vi "Get Experiments from PGserver.vi"(6 "conninfo":T2={"host"="localhost", "port"="5432", "client_encoding"="WIN1251", "dbname"="data", "user"="postgres", "password"=""}, 8 "error in (no error)":errorcluster, 9 "ParamColumns":string[](array[string])=["N", "Description"], 10 "ParamTable":string="experiments_1") -> (0 "error out":errorcluster, 2 "Names table":string[][](array[string]), 3 "Parameters table":dbl[][](array[numeric]))   [LabVIEW 2019, in "control.lvlib"]
uses:
  control.lvlib
  Database/ctl/Coninfo.ctl
  Database/PostgreSQL2LabVIEW/libpqlv/src/PQfinish.vi
  Database/PostgreSQL2LabVIEW/libpqlv/src/PQconnectdb.vi
  Database/PostgreSQL2LabVIEW/libpqlv/src/PQerrorMessage.vi
  Database/PostgreSQL2LabVIEW/libpqlv/src/PQstatus.vi
  <vilib>/dlg_ctls.llb/Space Constant.vi
  Database/PostgreSQL2LabVIEW/libpqUtility64/libpqutility64.lvlib
  Database/PostgreSQL2LabVIEW/libpqUtility/libpqutility.lvlib
  Database/PostgreSQL.lvlib
panel:
  out "PQStatus":T1(ring)
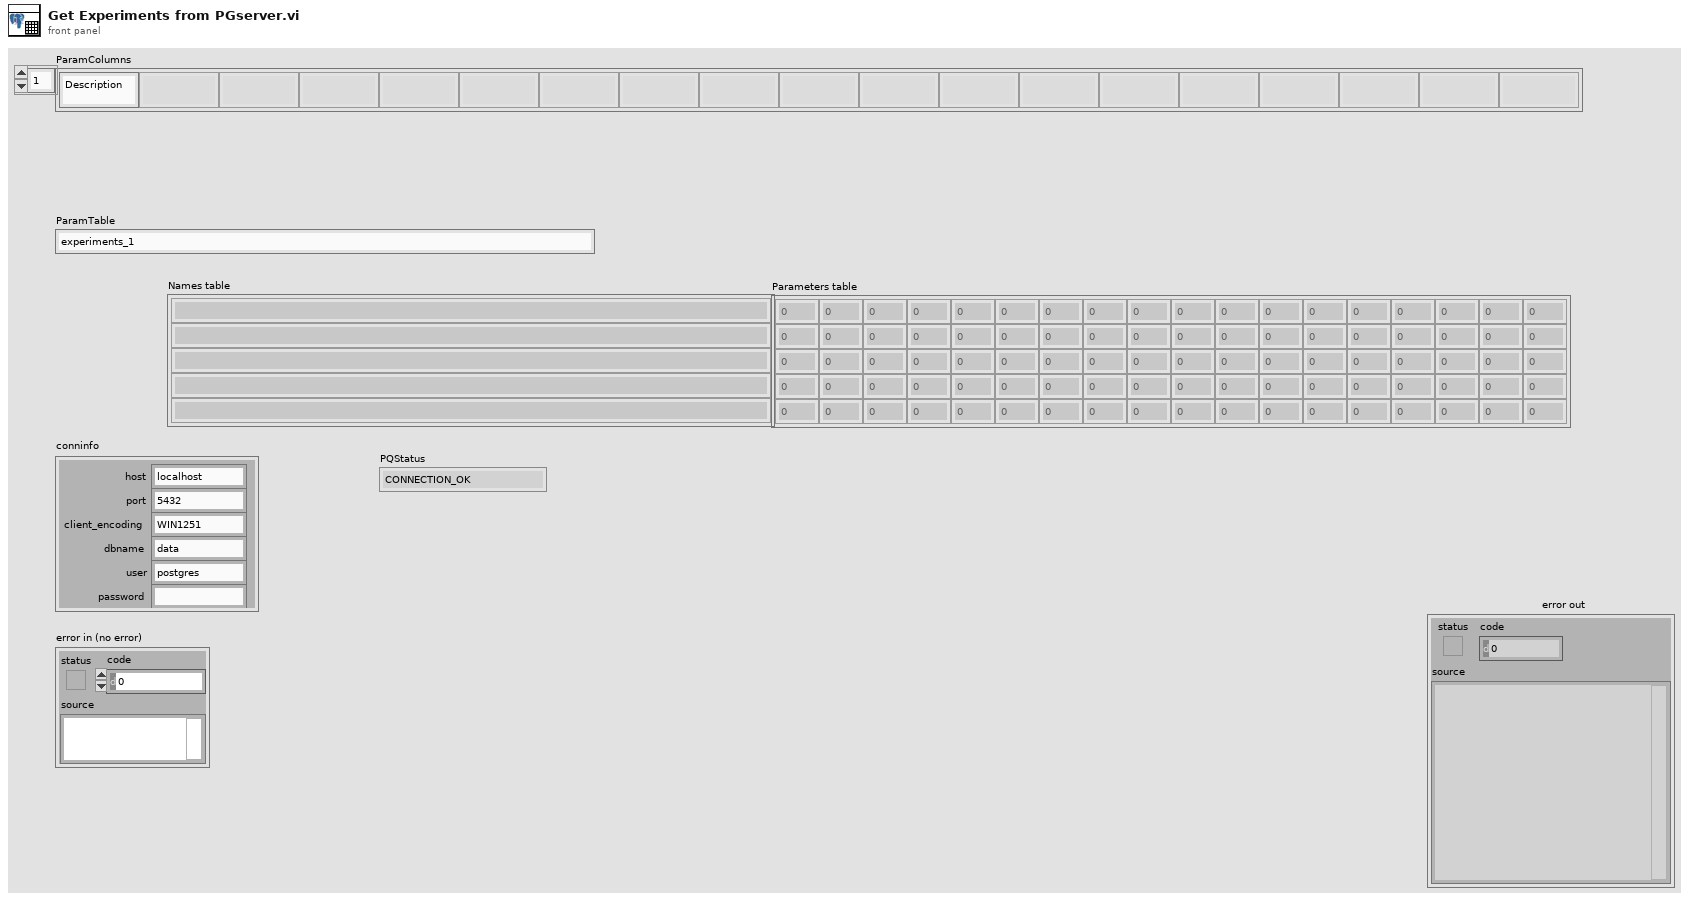
[diagram p1: front panel]
types:
  T1 = enum32{"CONNECTION_OK", "CONNECTION_BAD", "CONNECTION_STARTED", "CONNECTION_MADE", "CONNECTION_AWAITING_RESPONSE", "CONNECTION_AUTH_OK", "CONNECTION_SETENV", "CONNECTION_SSL_STARTUP", "CONNECTION_NEEDED"}
  T2 = typedef "PostgreSQL.lvlib/Coninfo.ctl" = cluster{"host":string, "port":string, "client_encoding":string, "dbname":string, "user":string, "password":string}
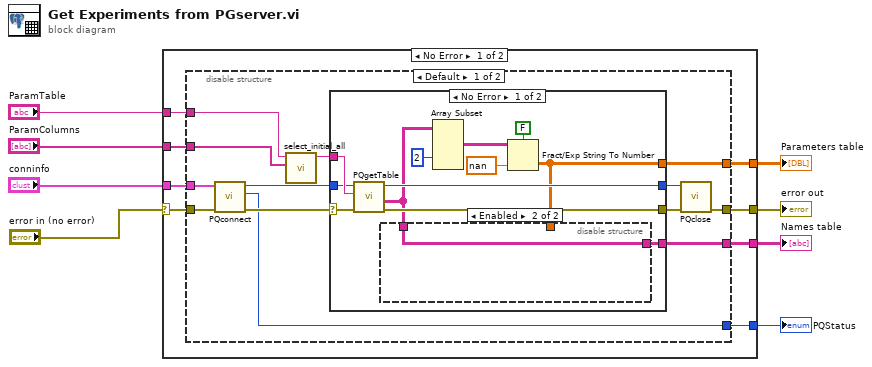
[diagram p0: block diagram]
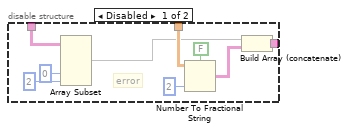
[diagram p2: hidden frame]
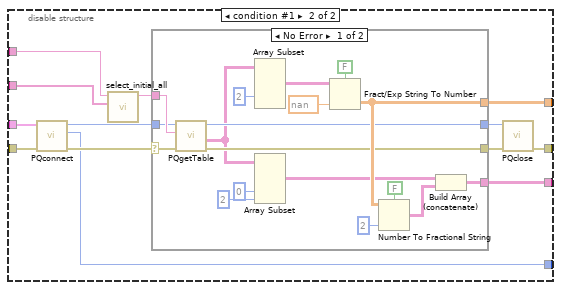
[diagram p4: hidden frame]
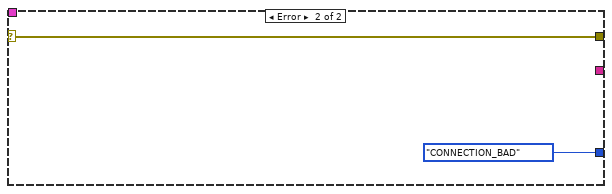
[diagram p6: hidden frame]
diagram:
  n1 = case shown="No Error" "error in (no error)" {
    selector: "error in (no error)" -> [w10 w88]
    tunnel: [w16 w88] -> w8
    tunnel: [w15 _] -> w7
    tunnel: [w14 _] -> w6
    tunnel: "ParamColumns" -> [w13 _]
    tunnel: "conninfo" -> [w12 _]
    tunnel: "ParamTable" -> [w11 _]
    tunnel: [w9 T1."CONNECTION_BAD" ("PQStatus")] -> w1
    frame No Error {
      n2 = disable-structure shown="Default" {
        disable-tunnel: [w18 w54] -> w16
        disable-tunnel: [w23 w63] -> w15
        disable-tunnel: [w22 w62] -> w14
        disable-tunnel: w13 -> [w17 w64]
        disable-tunnel: w12 -> [w26 w61]
        disable-tunnel: w11 -> [w24 w65]
        disable-tunnel: w10 -> [w25 w60]
        disable-tunnel: [w21 w57] -> w9
        frame condition #0 (active) {
          n3 = call "PQconnect.vi"("error in (no error)"=w25, "conninfo"=w26) -> ("error out"=w29:errorcluster, "PQStatus"=w21:T1, "conn"=w28:u32)  [unwired: 7 in]
          n4 = call "select_initial_all.vi"("Column table"=w17, "table"=w24) -> ("parameters"=w27:string)  [unwired: 8 in, 1 out]
          n5 = case shown="No Error" w29 {
            selector: w29 -> [w41 w53]
            tunnel: [w32 _] -> w23
            tunnel: [w30 _] -> w22
            tunnel: w28 -> [w39 w52]
            tunnel: w27 -> [w40 _]
            tunnel: [w37 w53] -> w19
            tunnel: [w38 w52] -> w20
            frame No Error {
              n6 = call "PQgetTable.vi"("error in"=w41, "query"=w40, "conn"=w39) -> ("error out"=w37:errorcluster, "Data"=w31:string[][], "conn_out"=w38:u32)  [unwired: 4 in, 2 out]
              n7 = Array Subset(array=w31, index (col)=2 ("index")) -> (w33:string[][])  [unwired: 3 in]
              n8 = Fract/Exp String To Number(use system decimal point (T)=FALSE, string=w33, default (0 dbl)=nan) -> (number=w32:dbl[][])  [unwired: 1 in, 1 out]
              n9 = disable-structure shown="Enabled" {
                disable-tunnel: w32 -> [w49 _]
                disable-tunnel: w31 -> [w47 w51]
                disable-tunnel: [w42 w51] -> w30
                frame Disabled {
                  # "error"
                  n10 = Array Subset(array=w47, index (col)=0 ("index"), length (col)=2 ("length")) -> (w44:string[][])  [unwired: 2 in]
                  n11 = Number To Fractional String(use system decimal point (T)=FALSE, number=w49, precision (6)=i16 2) -> (F-format string=w43:string[][])  [unwired: 1 in]
                  n12 = Build Array (concatenate)(w44, w43) -> (w42:string[][])
                }
                frame Enabled {
                }
              }
            }
            frame Error {
            }
          }
          n13 = call "PQclose.vi"("error in (no error)"=w19, "conn"=w20) -> ("error out"=w18:errorcluster)  [unwired: 9 in]
        }
        frame condition #1 {
          n14 = call "PQconnect.vi"("error in (no error)"=w60, "conninfo"=w61) -> ("error out"=w59:errorcluster, "PQStatus"=w57:T1, "conn"=w58:u64)  [unwired: 7 in]
          n15 = call "select_initial_all.vi"("Column table"=w64, "table"=w65) -> ("parameters"=w66:string)  [unwired: 8 in, 1 out]
          n16 = case shown="No Error" w59 {
            selector: w59 -> [w67 w86]
            tunnel: [w79 _] -> w63
            tunnel: [w73 _] -> w62
            tunnel: w58 -> [w68 w85]
            tunnel: w66 -> [w69 _]
            tunnel: [w71 w86] -> w55
            tunnel: [w72 w85] -> w56
            frame No Error {
              n17 = call "PQgetTable.vi"("error in"=w67, "query"=w69, "conn"=w68) -> ("error out"=w71:errorcluster, "Data"=w70:string[][], "conn_out"=w72:u64)  [unwired: 4 in, 2 out]
              n18 = Array Subset(array=w70, index (col)=2 ("index")) -> (w81:string[][])  [unwired: 3 in]
              n19 = Array Subset(array=w70, index (col)=0 ("index"), length (col)=2 ("length")) -> (w75:string[][])  [unwired: 2 in]
              n20 = Fract/Exp String To Number(use system decimal point (T)=FALSE, string=w81, default (0 dbl)=nan) -> (number=w79:dbl[][])  [unwired: 1 in, 1 out]
              n21 = Number To Fractional String(use system decimal point (T)=FALSE, number=w79, precision (6)=i16 2) -> (F-format string=w74:string[][])  [unwired: 1 in]
              n22 = Build Array (concatenate)(w75, w74) -> (w73:string[][])
            }
            frame Error {
            }
          }
          n23 = call "PQclose.vi"("error in (no error)"=w55, "conn"=w56) -> ("error out"=w54:errorcluster)  [unwired: 9 in]
        }
      }
    }
    frame Error {
    }
  }
  "error out" <- w8
  "Parameters table" <- w7
  "Names table" <- w6
  "PQStatus" <- w1
